vi "digital_gates.vi"() -> ()   [LabVIEW 2019]
panel:
  in  "input 2":bool
  in  "input 1":bool
  out ".not. (x .xor. y)?":bool
  out ".not. (x .or. y)?":bool
  out ".not. (x .and. y)?":bool
  out "x .xor. y?":bool
  out "x .or. y?":bool
  out "x .and. y?":bool
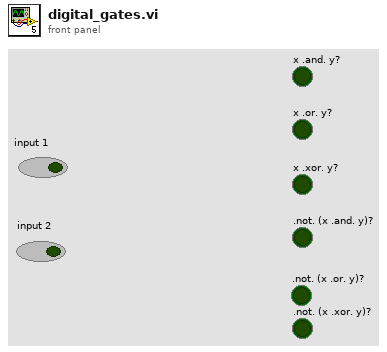
[diagram p1: front panel]
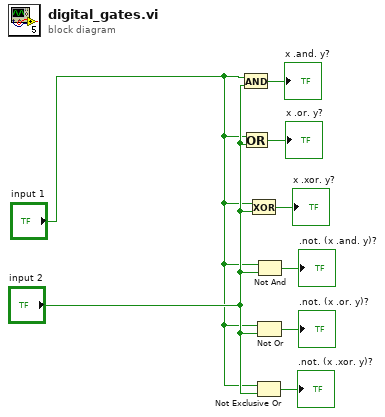
[diagram p0: block diagram]
diagram:
  n1 = And(x="input 1", y="input 2") -> (x .and. y?=→"x .and. y?":bool)
  n2 = Or(x="input 1", y="input 2") -> (x .or. y?=→"x .or. y?":bool)
  n3 = Exclusive Or(1:"input 2", 2:"input 1") -> (0:→"x .xor. y?":bool)
  n4 = Not Or(1:"input 2", 2:"input 1") -> (0:→".not. (x .or. y)?":bool)
  n5 = Not Exclusive Or(1:"input 2", 2:"input 1") -> (0:→".not. (x .xor. y)?":bool)
  n6 = Not And(1:"input 2", 2:"input 1") -> (0:→".not. (x .and. y)?":bool)
